vi "GetChanRunTime.vi"(8 "error in":errorcluster, 10 "Channel Number":T1=1 items=["Channel 1"=1, "Channel 2"=2, "Channel 3"=3, "Channel 4"=4, "Channel 5"=5, "Channel 6"=6, "Channel 7"=7, "Channel 8"=8], 11 "VISA resource name":refnum<visa-resource-name>) -> (0 "error out":errorcluster, 2 "channel run time":string, 3 "VISA resource name out":refnum<visa-resource-name>)   [LabVIEW 2023, in "Thermotron 8800.lvlib"]
doc: "CHRT\nCommand name: Channel run time\nCommand type: System status\nDescription: Queries the 8800 for a channel’s accumulated run time. The 8800 sends an integer to\nindicate the number of hours the channel has been running.\nSyntax: CHRTn?\nWhere n is any process variable channel (1 to 8).\nData type: Integer\nQuery example: CHRT2?\n8800 response: 962. This indicates that channel 2 has accumulated a total run time of 962 hours."
uses:
  Thermotron 8800.lvlib
  Private/AnalogInputChannelNumber.ctl
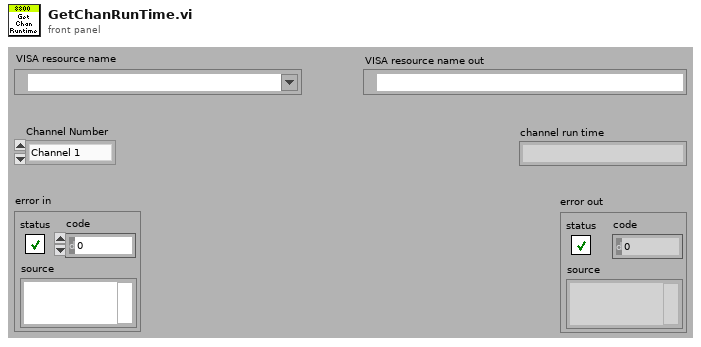
[diagram p1: front panel]
types:
  T1 = typedef "Thermotron 8800.lvlib/AnalogInputChannelNumber.ctl" = u16
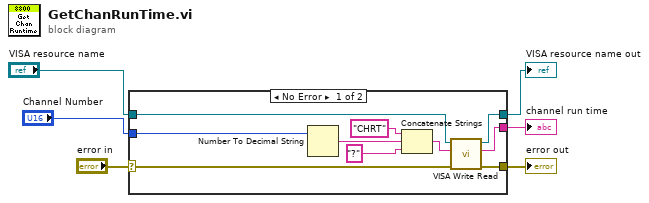
[diagram p0: block diagram]
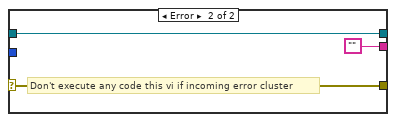
[diagram p2: hidden frame]
diagram:
  n1 = case shown="No Error" "error in" {
    selector: "error in" -> [w7 w19]
    tunnel: "Channel Number" -> [w12 _]
    tunnel: "VISA resource name" -> [w11 w18]
    tunnel: [w10 w19] -> w4
    tunnel: [w9 w18] -> w3
    tunnel: [w8 ""] -> w2
    frame No Error {
      n2 = Number To Decimal String(number=w12) -> (decimal integer string=w13:string)  [unwired: 1 in]
      n3 = Concatenate Strings("CHRT" ("8800 Command"), w13, "?" ("8800 Command")) -> (w14:string)
      n4 = call "VISA Write Read.vi"("error in (no error)"=w7, "8800 Command"=w14, "VISA Refnum in"=w11) -> ("error out"=w10:errorcluster, "read buffer"=w8:string, "VISA Refnum out"=w9:refnum<visa-resource-name>)  [unwired: 6 in]
    }
    frame Error {
      # "Don't execute any code this vi if incoming error cluster"
    }
  }
  "error out" <- w4
  "VISA resource name out" <- w3
  "channel run time" <- w2
